vi "LUnit Start Test.vi"(8 "error in (no error)":errorcluster, 10 "Tests":string[](array[string]), 11 "Coverage Report In":refnum<class "Coverage Report.lvclass">) -> (0 "error out":errorcluster, 3 "Coverage Report Out":refnum<class "Coverage Report.lvclass">)   [LabVIEW 2020, in "Coverage Report.lvclass"]
uses:
  Coverage Report.lvclass
  Coverage Report.lvclass/Coverage Report.ctl
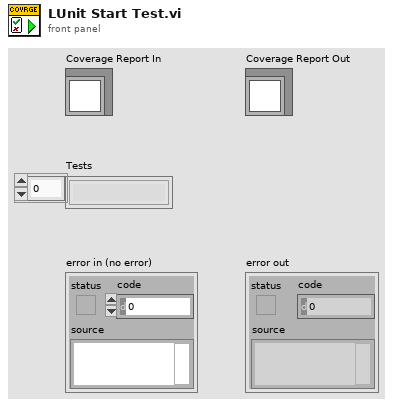
[diagram p1: front panel]
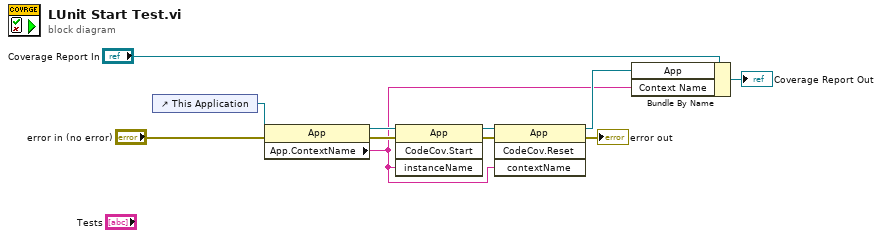
[diagram p0: block diagram]
diagram:
  n1 = control-ref of="This Application"() -> (w5:refnum<vi>)
  n2 = property class="App"(reference=w5, error in="error in (no error)") -> (reference out=w2:refnum<vi>, error out=w3:errorcluster, "App.ContextName"=w1:string)
  n3 = invoke class="App" method="CodeCov.Start"(reference=w2, error in=w3, "instanceName"=w1) -> (reference out=w7:refnum<vi>, error out=w6:errorcluster)  [unwired: 1 in, 2 out]
  n4 = invoke class="App" method="CodeCov.Reset"(reference=w7, error in=w6, "contextName"=w1) -> (reference out=w8:refnum<vi>, error out=→"error out":errorcluster)  [unwired: 1 in, 2 out]
  n5 = Bundle By Name(cluster="Coverage Report In", "App"=w8, "Context Name"=w1) -> (→"Coverage Report Out":refnum<class "Coverage Report.lvclass">)
